vi "UpdateIntegration.vi"(2 "error in (no error)":errorcluster, 4 "EpiWrapper in":refnum<class "EpiWrapper.lvclass">) -> (0 "error out":errorcluster, 1 "EpiWrapper out":refnum<class "EpiWrapper.lvclass">)   [LabVIEW 2012, in "EpiWrapper.lvclass"]
uses:
  EpiWrapper.lvclass
  EpiWrapper.lvclass/EpiWrapper.ctl
  Instruments.lvclass
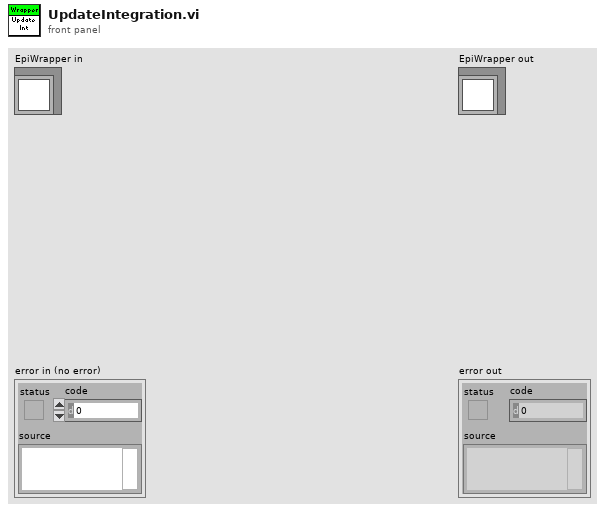
[diagram p1: front panel]
types:
  T1 = typedef "Config.ctl" = cluster{"IntTime":i32, "Samples":i32, "PowerMin":dbl, "KneeMin":dbl, "KneeMax":dbl}
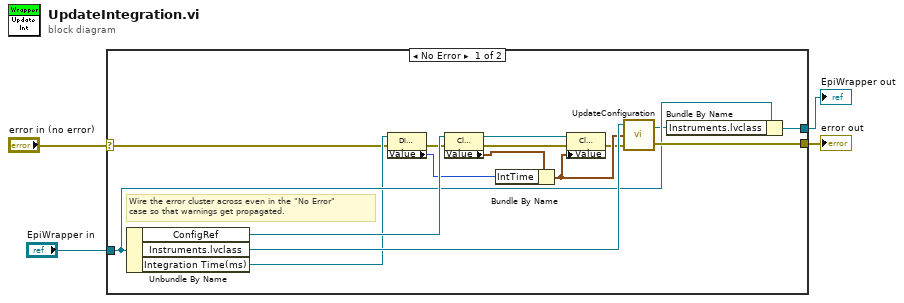
[diagram p0: block diagram]
diagram:
  n1 = case shown="No Error" "error in (no error)" {
    selector: "error in (no error)" -> [w5 w21]
    tunnel: [w12 w21] -> w3
    tunnel: [w9 w20] -> w1
    tunnel: "EpiWrapper in" -> [w11 w20]
    frame No Error {
      # "Wire the error cluster across even in the \"No Error\"\ncase so that warnings get propagated."
      n2 = Unbundle By Name(w11) -> ("ConfigRef"=w19:refnum<vi>, "Instruments.lvclass"=w15:refnum<class "Instruments.lvclass">, "Integration Time(ms)"=w8:refnum<vi>)
      n3 = property class="DigNum (strict)"(reference=w8, error in=w5) -> (error out=w6:errorcluster, "Value"=w7:i32)  [unwired: 1 out]
      n4 = property class="Clust (strict)"(reference=w19, error in=w6) -> (reference out=w17:refnum<vi>, error out=w16:errorcluster, "Value"=w18:T1)
      n5 = Bundle By Name(cluster=w18, "IntTime"=w7) -> (w14:T1)
      n6 = property class="Clust (strict)"(reference=w17, error in=w16, "Value"=w14) -> (error out=w13:errorcluster)  [unwired: 1 out]
      n7 = call-dynamic "UpdateConfiguration.vi"("error in (no error)"=w13, "ConfigIn"=w14, "Instruments in"=w15) -> ("error out"=w12:errorcluster, "Instruments out"=w10:refnum<class "Instruments.lvclass">)
      n8 = Bundle By Name(cluster=w11, "Instruments.lvclass"=w10) -> (w9:refnum<class "EpiWrapper.lvclass">)
    }
    frame Error {
    }
  }
  "error out" <- w3
  "EpiWrapper out" <- w1
